vi "MetadataFromRD.vi"(9 "ChannelNames":string[](array[string]), 10 "ChannelName":string, 11 "Raw data file":path) -> (1 "ValueStrings":string[](array[string]), 2 "ValueString":string)   [LabVIEW 2011]
panel:
  out "index of element 2":i32
  out "Name-Value Array":string[][](array[string])
  out "index of element":i32
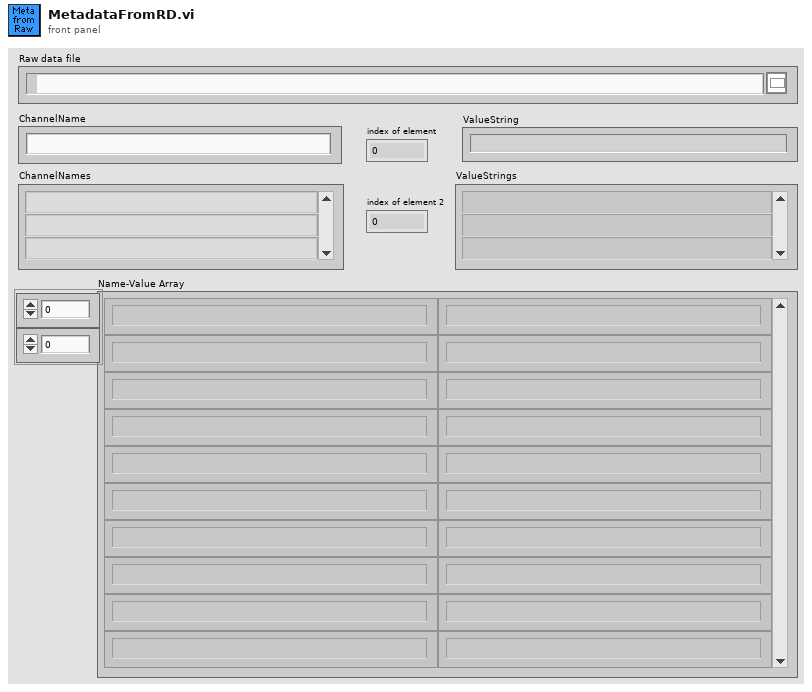
[diagram p1: front panel]
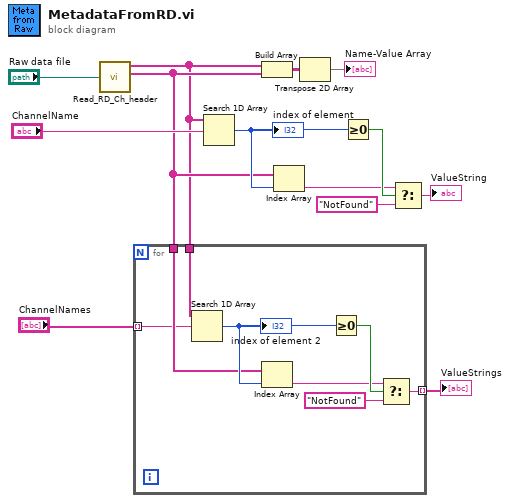
[diagram p0: block diagram]
diagram:
  n1 = call "Read_RD_Ch_header.vi"("Raw data file"="Raw data file") -> ("Ch Name Out"=w3:string[], "Ch Values"=w4:string[])  [unwired: 2 out]
  n2 = for {
    tunnel: w4 -> [w17]
    tunnel: w3 -> [w16]
    tunnel: "ChannelNames" -> [w15] mode=indexing
    tunnel: [w14] -> w1 mode=indexing
    n3 = Search 1D Array(1D array=w16, element=w15) -> (index of element=w21:i32)  [unwired: 1 in]
    "index of element 2" <- w21
    n4 = Index Array(array=w17, index=w21) -> (element=w19:string)
    n5 = Greater Or Equal To 0?(x=w21) -> (x >= 0?=w20:bool)
    n6 = Select(t=w19, s=w20, f="NotFound") -> (s? t:f=w14:string)
  }
  "ValueStrings" <- w1
  n7 = Search 1D Array(1D array=w3, element="ChannelName") -> (index of element=w9:i32)  [unwired: 1 in]
  "index of element" <- w9
  n8 = Build Array(w3, w4) -> (w11:string[][])
  n9 = Index Array(array=w4, index=w9) -> (element=w6:string)
  n10 = Transpose 2D Array(2D array=w11) -> (transposed array=→"Name-Value Array":string[][])
  n11 = Greater Or Equal To 0?(x=w9) -> (x >= 0?=w7:bool)
  n12 = Select(t=w6, s=w7, f="NotFound") -> (s? t:f=→"ValueString":string)
